vi "Teleop.vi"(10 "Match Info":T1={"Autonomous Elapsed Seconds"=0.0, "TeleOp Elapsed Seconds"=0.0, "Disabled Elapsed Seconds"=0.0, "Visited Autonomous"=FALSE, "Visited TeleOp"=FALSE, "Visited Disabled"=FALSE, "Autonomous Settings"={"Autonomous Style"=enum."Independent", "VI Refnum"=refnum}}, 11 "Call Context":T2) -> ()   [LabVIEW 2013]
doc: "This VI is called for each TeleOp packet received from the DS where the robot is not disabled. It is often used to read from the joysticks and update I/O or to update setpoints for timed control loops. It should complete and return within 20 milliseconds or it may miss DS packets."
uses:
  <vilib>/Rock Robotics/WPI/DriverStation/WPI_DriverStationDerivedRobotMode.ctl
  <vilib>/Rock Robotics/WPI/DriverStation/WPI_DriverStationMatch Info.ctl
  <vilib>/Rock Robotics/WPI/Solenoid/WPI_SolenoidValue.ctl
  Robot Global Data.vi
  <vilib>/Rock Robotics/WPI/Solenoid/Deprecated/WPI_SolenoidGetBool.vi
  <vilib>/Rock Robotics/WPI/Solenoid/WPI_SolenoidSetEnum.vi
  <vilib>/Rock Robotics/WPI/Joystick/WPI_JoystickGetSetRefNum.vi
  <vilib>/Rock Robotics/WPI/RobotDrive/WPI_RobotDriveGetSetRefNum.vi
panel:
  out "Numeric 1":dbl(slide) scale=0.0..100.0
  out "Boolean 2":bool
  out "Boolean 1":bool
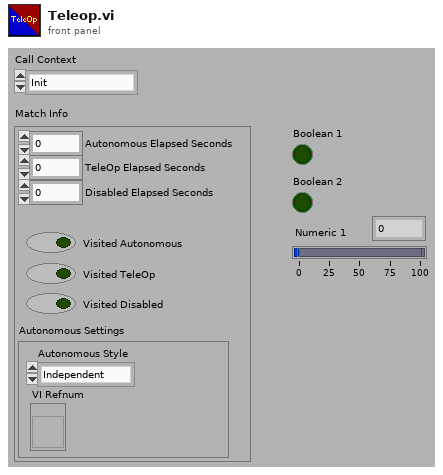
[diagram p1: front panel]
types:
  T1 = typedef "WPI_DriverStationMatch Info.ctl" = cluster{"Autonomous Elapsed Seconds":dbl, "TeleOp Elapsed Seconds":dbl, "Disabled Elapsed Seconds":dbl, "Visited Autonomous":bool, "Visited TeleOp":bool, "Visited Disabled":bool, "Autonomous Settings":cluster{"Autonomous Style":enum16{"Iterative", "Independent"}, "VI Refnum":refnum<vi>}}
  T2 = typedef "WPI_DriverStationDerivedRobotMode.ctl" = enum16{"Init", "Execute", "Stop"}
  T3 = typedef "WPI_RobotDriveDevRef.ctl" = cluster{"DevStatus":errorcluster, "Motors[]":T4[], "Square Inputs":bool, "Max Output":dbl, "Isochronous":bool}
  T4 = typedef "WPI_MotorControlDeviceRef.ctl" = cluster{"DeviceStatus":errorcluster, "Type":enum16{"PWM", "CAN"}, "PWM":cluster{"Digital Module":T5, "PWM Channel":T6, "DeadBand":T7}, "CAN":cluster{"Device Number":u8, "Control Mode":T8, "Semaphore":T9, "Max Vout":dbl}, "Invert":bool, "TransformRef":T10, "InvTransformRef":T10}
  T5 = typedef "FPGA_TypedefDigitalModule.ctl" = enum16{"Digital Module 1", "Digital Module 2"}
  T6 = typedef "FPGA_DIOPWMChannel.ctl" = enum8{"PWM 1", "PWM 2", "PWM 3", "PWM 4", "PWM 5", "PWM 6", "PWM 7", "PWM 8", "PWM 9", "PWM 10", "Invalid"}
  T7 = typedef "WPI_PWMDeadband.ctl" = cluster{"Name":string, "maxPositivePwm":i32, "minPositivePwm":i32, "centerPwm":i32, "maxNegativePwm":i32, "minNegativePwm":i32, "angularRange":u16}
  T8 = typedef "WPI_CANJaguar_ControlMode.ctl" = enum8{"Percent VBus", "Current", "Speed", "Position", "Voltage"}
  T9 = typedef "Semaphore RefNum" = refnum<k1>
  T10 = typedef "WPI_PWMTransform_ConPane.ctl" = refnum<vi>
  T11 = typedef "WPI_JoystickDevRef.ctl" = cluster{"Device":T12}
  T12 = typedef "WPI_JoystickDeviceEnum.ctl" = enum16{"USB 1", "USB 2", "USB 3", "USB 4", "Kinect 1", "Kinect 2"}
  T13 = typedef "WPI_JoystickButtonState.ctl" = cluster{"Button 1":bool, "Button 2":bool, "Button 3":bool, "Button 4":bool, "Button 5":bool, "Button 6":bool, "Button 7":bool, "Button 8":bool, "Button 9":bool, "Button 10":bool, "Button 11":bool, "Button 12":bool}
  T14 = cluster{"axis 1 (x)":dbl, "axis 2 (y)":dbl, "axis 3 (throttle)":dbl, "axis 4":dbl, "axis 5":dbl, "axis 6":dbl}
  T15 = typedef "WPI_AnalogChannelDevRef.ctl" = cluster{"DevStatus":errorcluster, "Analog Module":T16, "Analog Channel":T17}
  T16 = typedef "FPGA_TypedefAnalogModule.ctl" = enum16{"Analog Module 1", "Analog Module 2"}
  T17 = typedef "FPGA_AIChannel.ctl" = enum8{"AI 1", "AI 2", "AI 3", "AI 4", "AI 5", "AI 6", "AI 7", "AI 8", "Invalid"}
  T18 = typedef "WPI_RelayDevRef.ctl" = cluster{"DevStatus":errorcluster, "Relay Channel":T19, "Digital Module":T5, "Relay Direction":T20}
  T19 = typedef "FPGA_DIORelayChannel.ctl" = enum8{"Relay 1", "Relay 2", "Relay 3", "Relay 4", "Relay 5", "Relay 6", "Relay 7", "Relay 8", "Invalid"}
  T20 = typedef "WPI_RelayDirection.ctl" = enum16{"Both directions", "Forward only", "Reverse only"}
  T21 = typedef "WPI_SolenoidValue.ctl" = enum16{"Off", "On", "Forward", "Reverse"}
  T22 = typedef "WPI_SolenoidDevRef.ctl" = cluster{"DevStatus":errorcluster, "Solenoid Module":T23, "Forward Solenoid Channel":T24, "Reverse Solenoid Channel":T24}
  T23 = typedef "FPGA_TypedefSolenoidModule.ctl" = enum16{"Solenoid Module 1", "Solenoid Module 2"}
  T24 = typedef "WPI_SolenoidChannel.ctl" = enum8{"Solenoid 1", "Solenoid 2", "Solenoid 3", "Solenoid 4", "Solenoid 5", "Solenoid 6", "Solenoid 7", "Solenoid 8", "Invalid"}
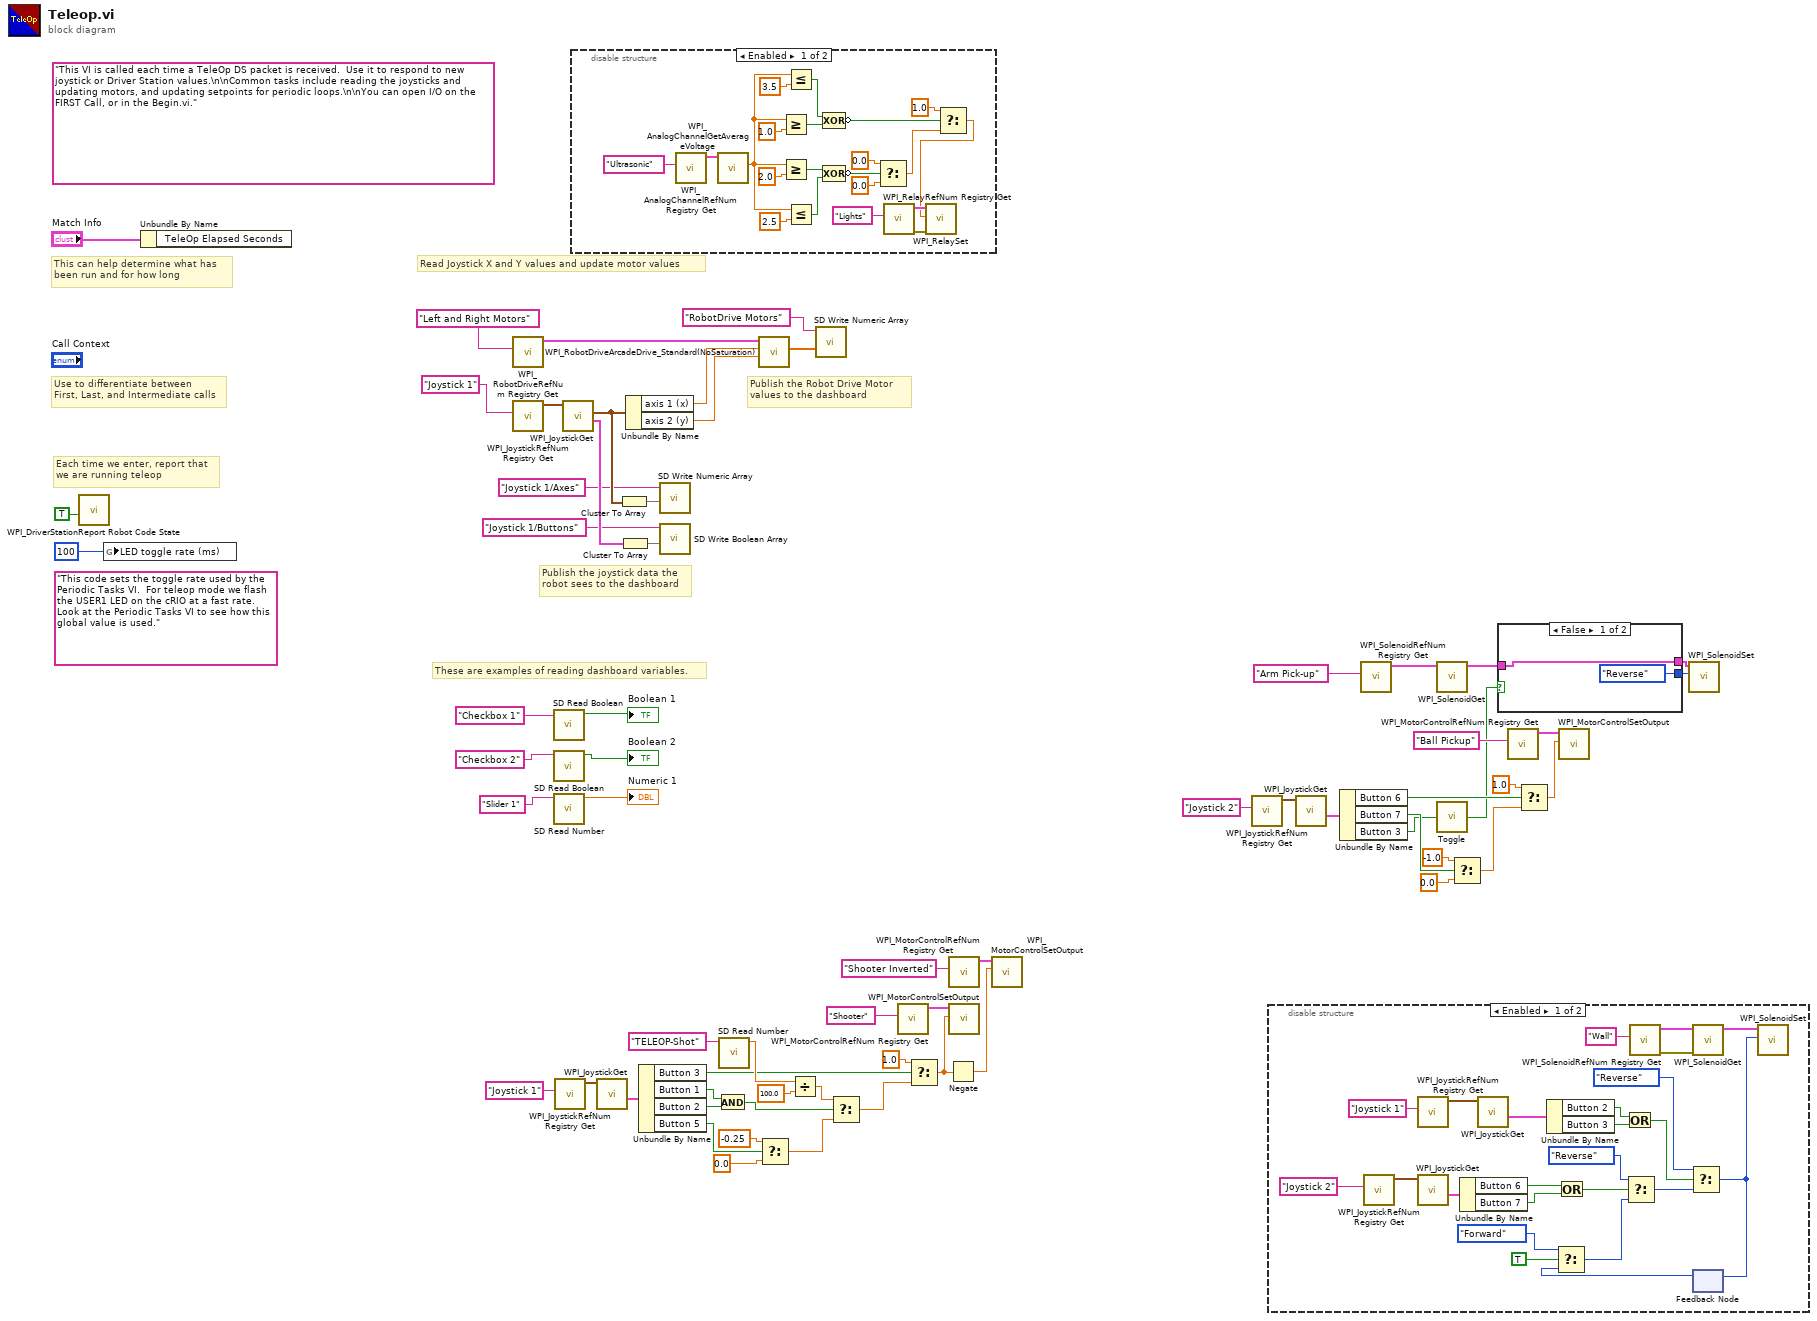
[diagram p0: block diagram]
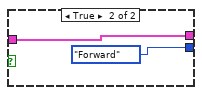
[diagram p4: hidden frame]
diagram:
  (unwired) "This code sets the toggle rate used by the Periodic Tasks VI.  For teleop mode we flash the USER1 LED on the cRIO at a fast rate.  Look at the Periodic Tasks VI to see how this global value is used."
  (unwired) "This VI is called each time a TeleOp DS packet is received.  Use it to respond to new joystick or Driver Station values.\n\nCommon tasks include reading the joysticks and updating motors, and updating setpoints for periodic loops.\n\nYou can open I/O on the FIRST Call, or in the Begin.vi."
  # "These are examples of reading dashboard variables."
  # "Publish the Robot Drive Motor\nvalues to the dashboard"
  # "Publish the joystick data the\nrobot sees to the dashboard"
  # "Each time we enter, report that\nwe are running teleop"
  # "Use to differentiate between\nFirst, Last, and Intermediate calls"
  # "This can help determine what has\nbeen run and for how long"
  # "Read Joystick X and Y values and update motor values"
  n1 = call <vilib>:"WPI_DriverStationReport Robot Code State.vi"("TeleOp"=TRUE ("Autonomous")) -> ()  [unwired: 10 in, 1 out]
  n2 = global write "Robot Global Data.vi" "LED toggle rate (ms)"(u32 100 ("LED ms toggle rate")) -> ()
  n3 = Unbundle By Name("Match Info") -> ()  [unwired: 1 out]
  n4 = call <vilib>:"WPI_RobotDriveRefNum Registry Get.vi"("refnum name"="Left and Right Motors") -> ("RobotDriveDevRef"=w63:T3)  [unwired: 1 in, 9 out]
  n5 = call <vilib>:"WPI_JoystickRefNum Registry Get.vi"("refnum name"="Joystick 1") -> ("JoystickDevRef"=w59:T11)  [unwired: 1 in, 9 out]
  n6 = call <vilib>:"SD Read Boolean.vi"("Name"="Checkbox 1" ("refnum name")) -> ("Boolean"=→"Boolean 1":bool)  [unwired: 8 in, 2 out]
  n7 = call <vilib>:"SD Read Boolean.vi"("Name"="Checkbox 2" ("refnum name")) -> ("Boolean"=→"Boolean 2":bool)  [unwired: 8 in, 2 out]
  n8 = call <vilib>:"SD Read Number.vi"("Name"="Slider 1" ("refnum name")) -> ("Numeric"=→"Numeric 1":dbl)  [unwired: 8 in, 2 out]
  n9 = call <vilib>:"WPI_JoystickRefNum Registry Get.vi"("refnum name"="Joystick 1") -> ("JoystickDevRef"=w41:T11)  [unwired: 1 in, 9 out]
  n10 = call <vilib>:"WPI_JoystickGet.vi"("JoystickDevRef"=w59) -> ("Buttons"=w56:T13, "Axes"=w53:T14)  [unwired: 1 in, 4 out]
  n11 = disable-structure shown="Enabled" {
    frame Enabled {
      n12 = call <vilib>:"WPI_AnalogChannelRefNum Registry Get.vi"("refnum name"="Ultrasonic") -> ("AIDeviceRef"=w85:T15)  [unwired: 9 in, 1 out]
      n13 = call <vilib>:"WPI_AnalogChannelGetAverageVoltage.vi"("AIDeviceRef"=w85) -> ("Voltage"=w76:dbl)  [unwired: 8 in, 2 out]
      n14 = Greater Or Equal?(x=w76, y=1.0) -> (x >= y?=w79:bool)
      n15 = Greater Or Equal?(x=w76, y=2.0) -> (x >= y?=w73:bool)
      n16 = Less Or Equal?(x=w76, y=3.5) -> (x <= y?=w78:bool)
      n17 = Less Or Equal?(x=w76, y=2.5) -> (x <= y?=w74:bool)
      n18 = Compound Arithmetic op=XOR(w78, w79) -> (invert w71:bool)
      n19 = Compound Arithmetic op=XOR(w73, w74) -> (invert w72:bool)
      n20 = Select(t=0.0, s=w72, f=0.0) -> (s? t:f=w67:dbl)
      n21 = call <vilib>:"WPI_RelayRefNum Registry Get.vi"("refnum name"="Lights") -> ("error out"=w84:errorcluster, "RelayDevRef"=w83:T18)  [unwired: 9 in]
      n22 = Select(t=1.0, s=w71, f=w67) -> (s? t:f=w66:dbl)
      n23 = call <vilib>:"WPI_RelaySet.vi"("error in (no error)"=w84, "RelayValue"=w66, "RelayDevRef"=w83) -> ()  [unwired: 7 in, 2 out]
    }
    frame Disabled {
    }
  }
  n24 = call <vilib>:"WPI_JoystickGet.vi"("JoystickDevRef"=w41) -> ("Buttons"=w40:T13)  [unwired: 1 in, 5 out]
  n25 = Cluster To Array(cluster=w53) -> (array=w52:dbl[])
  n26 = Cluster To Array(cluster=w56) -> (array=w55:bool[])
  n27 = Unbundle By Name(w53) -> ("axis 1 (x)"=w62:dbl, "axis 2 (y)"=w61:dbl)
  n28 = Unbundle By Name(w40) -> ("Button 3"=w4:bool, "Button 1"=w9:bool, "Button 2"=w10:bool, "Button 5"=w38:bool)
  n29 = call <vilib>:"SD Write Numeric Array.vi"("Numeric Array"=w52, "Name"="Joystick 1/Axes") -> ()  [unwired: 8 in, 2 out]
  n30 = call <vilib>:"SD Write Boolean Array.vi"("Boolean Array"=w55, "Name"="Joystick 1/Buttons") -> ()  [unwired: 8 in, 2 out]
  n31 = And(x=w9, y=w10) -> (x .and. y?=w39:bool)
  n32 = call <vilib>:"SD Read Number.vi"("Name"="TELEOP-Shot") -> ("Numeric"=w7:dbl)  [unwired: 8 in, 2 out]
  n33 = call <vilib>:"WPI_RobotDriveArcadeDrive_Standard(NoSaturation).vi"("Y axis value"=w61, "X axis value"=w62, "RobotDriveDevRef"=w63) -> ("Motor Values"=w49:dbl[])  [unwired: 1 in, 7 out]
  n34 = Select(t=-0.25, s=w38, f=0.0) -> (s? t:f=w35:dbl)
  n35 = Divide(x=w7, y=100.0) -> (x/y=w5:dbl)
  n36 = call <vilib>:"SD Write Numeric Array.vi"("Numeric Array"=w49, "Name"="RobotDrive Motors") -> ()  [unwired: 8 in, 2 out]
  n37 = Select(t=w5, s=w39, f=w35) -> (s? t:f=w3:dbl)
  n38 = call <vilib>:"WPI_MotorControlRefNum Registry Get.vi"("refnum name"="Shooter") -> ("MotorControlDevRef"=w33:T4)  [unwired: 9 in, 1 out]
  n39 = Select(t=1.0, s=w4, f=w3) -> (s? t:f=w1:dbl)
  n40 = Negate(x=w1) -> (-x=w31:dbl)
  n41 = call <vilib>:"WPI_MotorControlRefNum Registry Get.vi"("refnum name"="Shooter Inverted") -> ("MotorControlDevRef"=w30:T4)  [unwired: 9 in, 1 out]
  n42 = call <vilib>:"WPI_MotorControlSetOutput.vi"("Output"=w1, "MotorControlDevRef"=w33) -> ()  [unwired: 7 in, 3 out]
  n43 = call <vilib>:"WPI_MotorControlSetOutput.vi"("Output"=w31, "MotorControlDevRef"=w30) -> ()  [unwired: 7 in, 3 out]
  n44 = call <vilib>:"WPI_JoystickRefNum Registry Get.vi"("refnum name"="Joystick 2") -> ("JoystickDevRef"=w29:T11)  [unwired: 1 in, 9 out]
  n45 = disable-structure shown="Enabled" {
    frame Enabled {
      n46 = call <vilib>:"WPI_JoystickRefNum Registry Get.vi"("refnum name"="Joystick 2") -> ("JoystickDevRef"=w110:T11)  [unwired: 9 in, 1 out]
      n47 = call <vilib>:"WPI_JoystickRefNum Registry Get.vi"("refnum name"="Joystick 1") -> ("JoystickDevRef"=w109:T11)  [unwired: 9 in, 1 out]
      n48 = call <vilib>:"WPI_JoystickGet.vi"("JoystickDevRef"=w110) -> ("Buttons"=w105:T13)  [unwired: 4 in, 2 out]
      n49 = Unbundle By Name(w105) -> ("Button 6"=w92:bool, "Button 7"=w91:bool)
      n50 = call <vilib>:"WPI_JoystickGet.vi"("JoystickDevRef"=w109) -> ("Buttons"=w106:T13)  [unwired: 4 in, 2 out]
      n51 = Unbundle By Name(w106) -> ("Button 2"=w89:bool, "Button 3"=w88:bool)
      n52 = Or(x=w92, y=w91) -> (x .or. y?=w90:bool)
      n53 = Or(x=w89, y=w88) -> (x .or. y?=w87:bool)
      n54 = call <vilib>:"WPI_SolenoidRefNum Registry Get.vi"("refnum name"="Wall") -> ("error out"=w96:errorcluster, "SolenoidDevRef"=w97:T22)  [unwired: 9 in]
      n55 = call-poly <vilib>:"WPI_SolenoidGet.vi"("error in (no error)"=w96, "SolenoidDevRef"=w97) -> ("SolenoidDevRef"=w95:T22)  [unwired: 7 in, 2 out]
      n56 = feedback #1() -> (w93:T21)  [unwired: 1 in]
      n57 = Select(t=WPI_SolenoidValue."Forward" ("Value"), s=TRUE, f=w93) -> (s? t:f=w100:T21)
      n58 = Select(t=WPI_SolenoidValue."Reverse" ("Value"), s=w90, f=w100) -> (s? t:f=w99:T21)
      n59 = Select(t=WPI_SolenoidValue."Reverse" ("Value"), s=w87, f=w99) -> (s? t:f=w94:T21)
      n60 = feedback-in #1(w94) -> ()
      n61 = call-poly <vilib>:"WPI_SolenoidSet.vi"("Value"=w94, "SolenoidDevRef"=w95) -> ()  [unwired: 8 in, 2 out]
    }
    frame Disabled {
    }
  }
  n62 = call <vilib>:"WPI_JoystickGet.vi"("JoystickDevRef"=w29) -> ("Buttons"=w27:T13)  [unwired: 1 in, 5 out]
  n63 = Unbundle By Name(w27) -> ("Button 6"=w25:bool, "Button 7"=w26:bool, "Button 3"=w17:bool)
  n64 = call <vilib>:"WPI_SolenoidRefNum Registry Get.vi"("refnum name"="Arm Pick-up") -> ("SolenoidDevRef"=w15:T22)  [unwired: 9 in, 1 out]
  n65 = call-poly <vilib>:"WPI_SolenoidGet.vi"("SolenoidDevRef"=w15) -> ("SolenoidDevRef"=w14:T22)  [unwired: 8 in, 2 out]
  n66 = call "Toggle.vi"("Input"=w17) -> ("Toggled Output"=w16:bool)
  n67 = Select(t=-1.0, s=w26, f=0.0) -> (s? t:f=w21:dbl)
  n68 = case shown="False" w16 {
    tunnel: w14 -> [w112 w114]
    tunnel: [w112 w114] -> w12
    tunnel: [WPI_SolenoidValue."Reverse" ("Value") WPI_SolenoidValue."Forward" ("Value")] -> w11
    frame False {
    }
    frame True {
    }
  }
  n69 = call <vilib>:"WPI_MotorControlRefNum Registry Get.vi"("refnum name"="Ball Pickup") -> ("MotorControlDevRef"=w19:T4)  [unwired: 9 in, 1 out]
  n70 = Select(t=1.0, s=w25, f=w21) -> (s? t:f=w18:dbl)
  n71 = call <vilib>:"WPI_MotorControlSetOutput.vi"("Output"=w18, "MotorControlDevRef"=w19) -> ()  [unwired: 7 in, 3 out]
  n72 = call-poly <vilib>:"WPI_SolenoidSet.vi"("Value"=w11, "SolenoidDevRef"=w12) -> ()  [unwired: 8 in, 2 out]
